vi "Save File Check For Old Summary File.vi"(8 "Error In":errorcluster, 10 "Summary":string, 11 "Path in":path) -> (0 "Error Out":errorcluster, 2 "New Summary Created":bool, 3 "Path out":path)   [LabVIEW 2020, in "Save File.lvlib"]
uses:
  Save File.lvlib
panel:
  out "Filename List":string[](array[string])
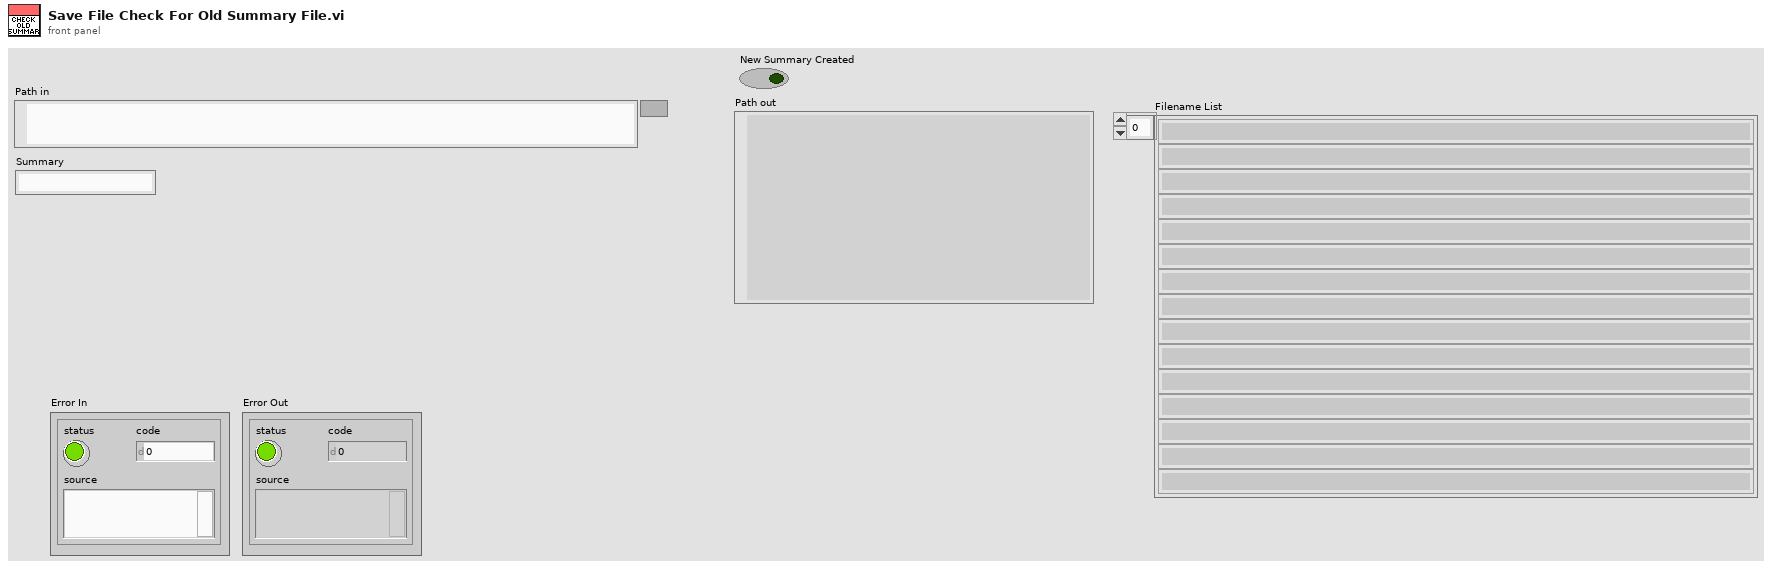
[diagram p1: front panel]
types:
  T1 = enum16{"open", "replace", "create", "open or create", "replace or create", "replace or create with confirmation"}
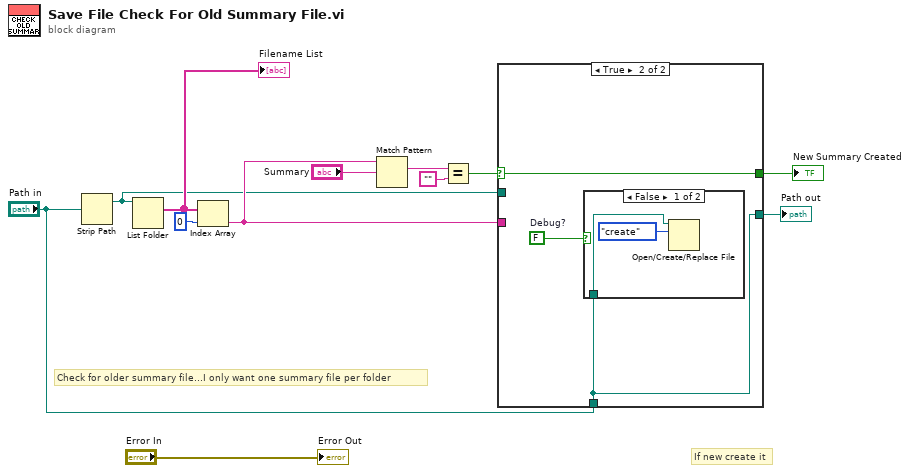
[diagram p0: block diagram]
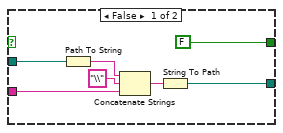
[diagram p2: hidden frame]
diagram:
  # "If new create it"
  # "Check for older summary file...I only want one summary file per folder"
  n1 = Strip Path(path="Path in") -> (stripped path=w4:path)  [unwired: 1 out]
  n2 = List Folder(path=w4) -> (filenames=w11:string[])  [unwired: 3 in, 3 out]
  "Filename List" <- w11
  n3 = Index Array(array=w11, index=0) -> (element=w5:string)
  n4 = Match Pattern(string=w5, regular expression="Summary") -> (match substring=w8:string)  [unwired: 1 in, 3 out]
  n5 = Equal?(x=w8, y="") -> (x = y?=w6:bool)
  n6 = case shown="True" w6 {
    selector: w6 -> [_ w21]
    tunnel: "Path in" -> [_ w22]
    tunnel: w5 -> [w18 _]
    tunnel: [w19 w22] -> w3
    tunnel: w4 -> [w16 _]
    tunnel: [FALSE w21] -> w2
    frame False {
      n7 = Path To String(path=w16) -> (string=w15:string)
      n8 = Concatenate Strings(w15, "\\" ("string"), w18) -> (w14:string)
      n9 = String To Path(string=w14) -> (path=w19:path)
    }
    frame True {
      w20 = FALSE  # Debug?
      n10 = case shown="False" w20 {
        tunnel: w22 -> [w23 _]
        frame False {
          n11 = Open/Create/Replace File(file path (use dialog)=w23, operation (0:open)=T1."create") -> ()  [unwired: 4 in, 3 out]
        }
        frame True {
        }
      }
    }
  }
  "Path out" <- w3
  "New Summary Created" <- w2
  "Error Out" <- "Error In"
